vi "Read Key (Path).vi"(7 "section":string, 8 "error in (no error)":errorcluster, 9 "default value":path, 10 "key":string, 11 "refnum":T1) -> (0 "error out":errorcluster, 1 "value":path, 2 "found?":bool, 3 "refnum out":T1)   [LabVIEW 2009]
doc: "Reads a value associated with a key in a specified section from the configuration data identified by <B>refnum</B>. If the key does not exist, the VI returns the default value. You can use this polymorphic VI to read the following types of values from a key: Boolean, double-precision numeric, signed integer, path, string, and unsigned integer. The data type you wire to the <B>default value</B> input determines the polymorphic instance to use."
uses:
  <vilib>/Utility/config.llb/Config Data RefNum.ctl
  <vilib>/Utility/config.llb/NI_LVConfig.lvlib
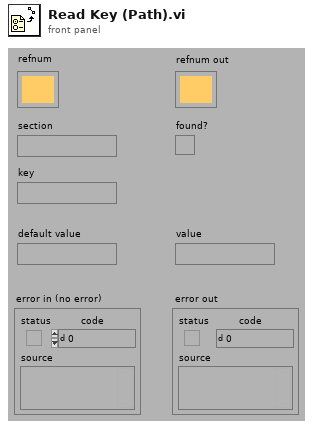
[diagram p1: front panel]
types:
  T1 = typedef "NI_LVConfig.lvlib/Config Data RefNum.ctl" = refnum<k1>
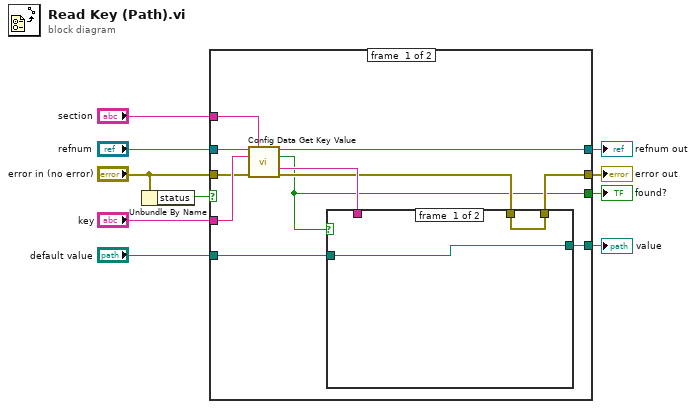
[diagram p0: block diagram]
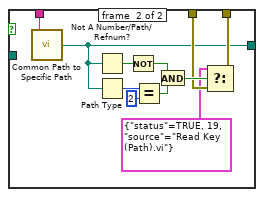
[diagram p2: hidden frame]
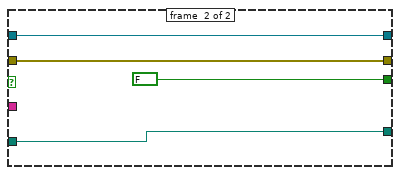
[diagram p3: hidden frame]
diagram:
  n1 = Unbundle By Name("error in (no error)") -> ("status"=w10:bool)
  n2 = case shown="False" w10 {
    tunnel: [w19 w37] -> w8
    tunnel: [w12 w38] -> w7
    tunnel: "refnum" -> [w16 w37]
    tunnel: "error in (no error)" -> [w17 w38]
    tunnel: "section" -> [w21 _]
    tunnel: "key" -> [w20 _]
    tunnel: [w11 FALSE ("section exists?")] -> w6
    tunnel: [w14 w36] -> w9
    tunnel: "default value" -> [w15 w36]
    frame #0 {
      n3 = call "Config Data Get Key Value.vi"("config data"=w16, "section"=w21, "key"=w20, "error in (no error)"=w17) -> ("config data out"=w19:T1, "key exists?"=w11:bool, "key value"=w18:string, "error out"=w13:errorcluster)  [unwired: 6 in, 2 out]
      n4 = case shown="True" w11 {
        tunnel: w18 -> [_ w34]
        tunnel: w15 -> [w23 _]
        tunnel: [w23 w24] -> w14
        tunnel: w13 -> [w22 w27]
        tunnel: [w22 w26] -> w12
        frame #0 {
        }
        frame #1 {
          n5 = call "Common Path to Specific Path.vi"("common path"=w34) -> ("specific path"=w24:path)  [unwired: 4 in]
          n6 = Not A Number/Path/Refnum?(number/path/refnum=w24) -> (NaN/Path/Refnum?=w31:bool)
          n7 = Path Type(1:w24) -> (0:w33:i16)
          n8 = Not(x=w31) -> (.not. x?=w30:bool)
          n9 = Equal?(x=w33, y=i16 2) -> (x = y?=w29:bool)
          n10 = And(x=w30, y=w29) -> (x .and. y?=w28:bool)
          n11 = Select(t=cluster{"status":bool, u16, "source":string} {"status"=TRUE, 19, "source"="Read Key (Path).vi"} ("f"), s=w28, f=w27) -> (s? t:f=w26:errorcluster)
        }
      }
    }
    frame #1 {
    }
  }
  "error out" <- w7
  "refnum out" <- w8
  "value" <- w9
  "found?" <- w6
